vi "Set Mode.vi"(0 "CS.lvclass in":refnum<class "CS.lvclass">, 1 "On&G 0":T1, 2 "On&G 1":T1, 3 "On&G 2":T1, 4 "On&G 3":T1, 5 "error in (no error)":errorcluster) -> (14 "CS.lvclass out":refnum<class "CS.lvclass">, 19 "error out":errorcluster)   [LabVIEW 2016, in "CS.lvclass"]
uses:
  Lib.llb/CS.lvclass
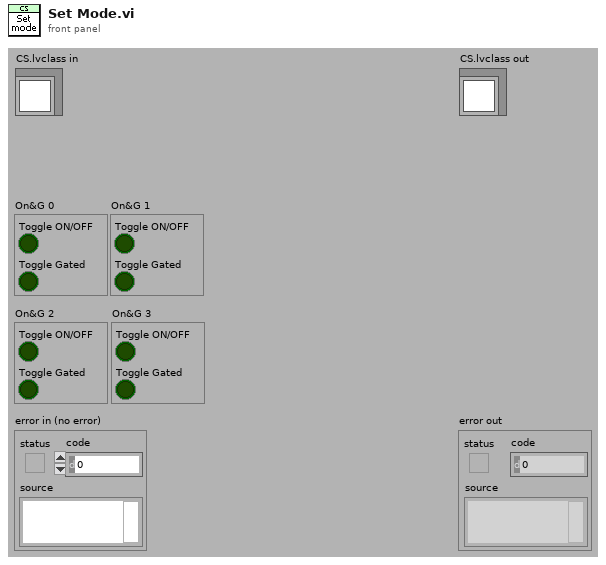
[diagram p1: front panel]
types:
  T1 = cluster{"Toggle ON/OFF":bool, "Toggle Gated":bool}
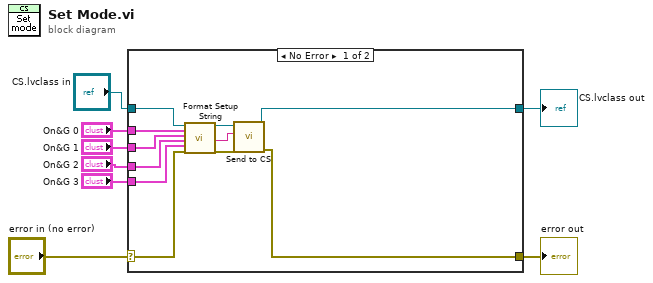
[diagram p0: block diagram]
diagram:
  n1 = case shown="No Error" "error in (no error)" {
    selector: "error in (no error)" -> [w15 w20]
    tunnel: [w14 w20] -> w7
    tunnel: [w19 w21] -> w5
    tunnel: "CS.lvclass in" -> [w17 w21]
    tunnel: "On&G 3" -> [w12 _]
    tunnel: "On&G 2" -> [w11 _]
    tunnel: "On&G 1" -> [w10 _]
    tunnel: "On&G 0" -> [w9 _]
    frame No Error {
      n2 = call-dynamic "Format Setup String.vi"("CS in"=w17, "On&G 0"=w9, "On&G 1"=w10, "On&G 2"=w11, "On&G 3"=w12, "error in (no error)"=w15) -> ("CS out"=w18:refnum<class "CS.lvclass">, "Setup string"=w13:string, "error out"=w16:errorcluster)  [unwired: 11 in]
      n3 = call-dynamic "Send to CS.vi"("error in (no error)"=w16, "String to write"=w13, "CS in"=w18) -> ("error out"=w14:errorcluster, "CS out"=w19:refnum<class "CS.lvclass">)  [unwired: 7 in]
    }
    frame Error {
    }
  }
  "error out" <- w7
  "CS.lvclass out" <- w5
